vi "bh3_get_battery_status.vi"(8 "error in (no error)":errorcluster, 11 "bt connection ID in":refnum<k31>) -> (0 "error out":errorcluster, 1 "voltage(mv)":u16, 2 "change (%)":u8, 3 "bt connection ID out":refnum<k31>)   [LabVIEW 2013]
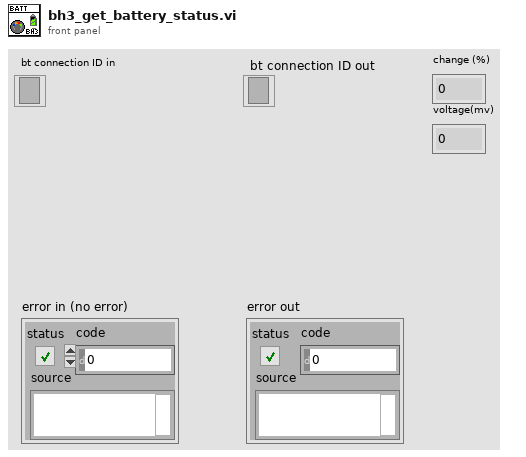
[diagram p1: front panel]
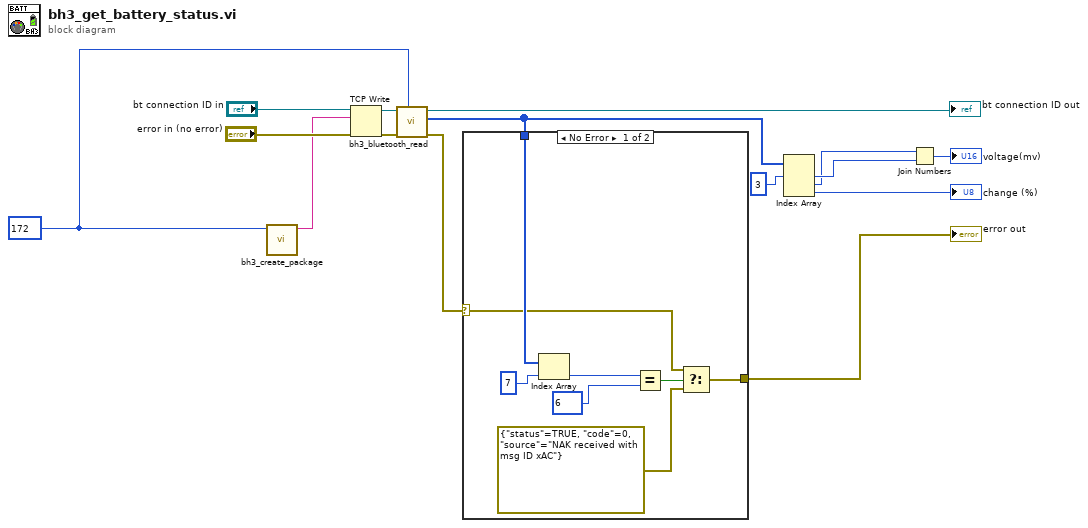
[diagram p0: block diagram]
diagram:
  w7 = u8 172 ("msg_ID")
  n1 = call "bh3_create_package.vi"("msg_ID"=w7) -> ("package string"=w13:string)  [unwired: 9 in, 1 out]
  n2 = TCP Write(connection ID="bt connection ID in", data in=w13, error in (no error)="error in (no error)") -> (connection ID out=w10:refnum<k31>, error out=w12:errorcluster)  [unwired: 1 in, 1 out]
  n3 = call "bh3_bluetooth_read.vi"("command_expected(x00)"=w7, "error in (no error)"=w12, "bt connection ID in"=w10) -> ("error out"=w8:errorcluster, "response byte array"=w6:u8[], "bt connection ID out"=→"bt connection ID out":refnum<k31>)  [unwired: 6 in]
  n4 = case shown="No Error" w8 {
    selector: w8 -> [w16 w24]
    tunnel: w6 -> [w23 _]
    tunnel: [w18 w24] -> w9
    frame No Error {
      n5 = Index Array(array=w23, index=7) -> (element=w21:u8)
      n6 = Equal?(x=w21, y=u8 6 ("msg_ID")) -> (x = y?=w19:bool)
      n7 = Select(t=w16, s=w19, f=errorcluster {"status"=TRUE, "code"=0, "source"="NAK received with msg ID xAC"} ("s? t:f")) -> (s? t:f=w18:errorcluster)
    }
    frame Error {
    }
  }
  "error out" <- w9
  n8 = Index Array(array=w6, index #1=3 ("index")) -> (element #1=w4:u8, element #2=w3:u8, element #3=→"change (%)":u8)  [unwired: 2 in]
  n9 = Join Numbers(hi=w3, lo=w4) -> ((hi.lo)=→"voltage(mv)":u16)
